vi "Disabled - Data Logger (SubVI).vi"(4 "Data Acquisition Array":string[][](array[string]), 7 "Header Names Input":string[](array[string]), 8 "File Index In":i32, 9 "was teleop Input?":bool, 10 "File Name":string, 11 "Path":string="/home/lvuser/Data/") -> (0 "File Index Out":i32, 2 "File Name Out":string, 3 "Was in Teleop Ouput?":bool)   [LabVIEW 2019]
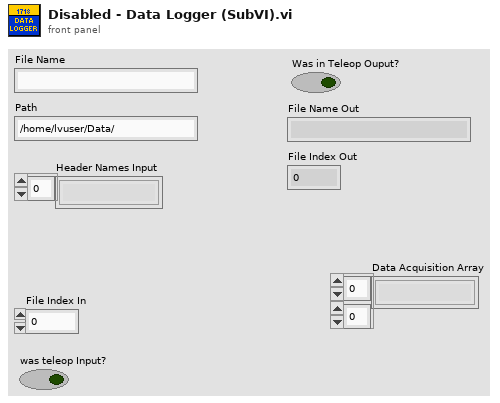
[diagram p1: front panel]
types:
  T1 = enum16{"open", "replace", "create", "open or create", "replace or create", "replace or create with confirmation"}
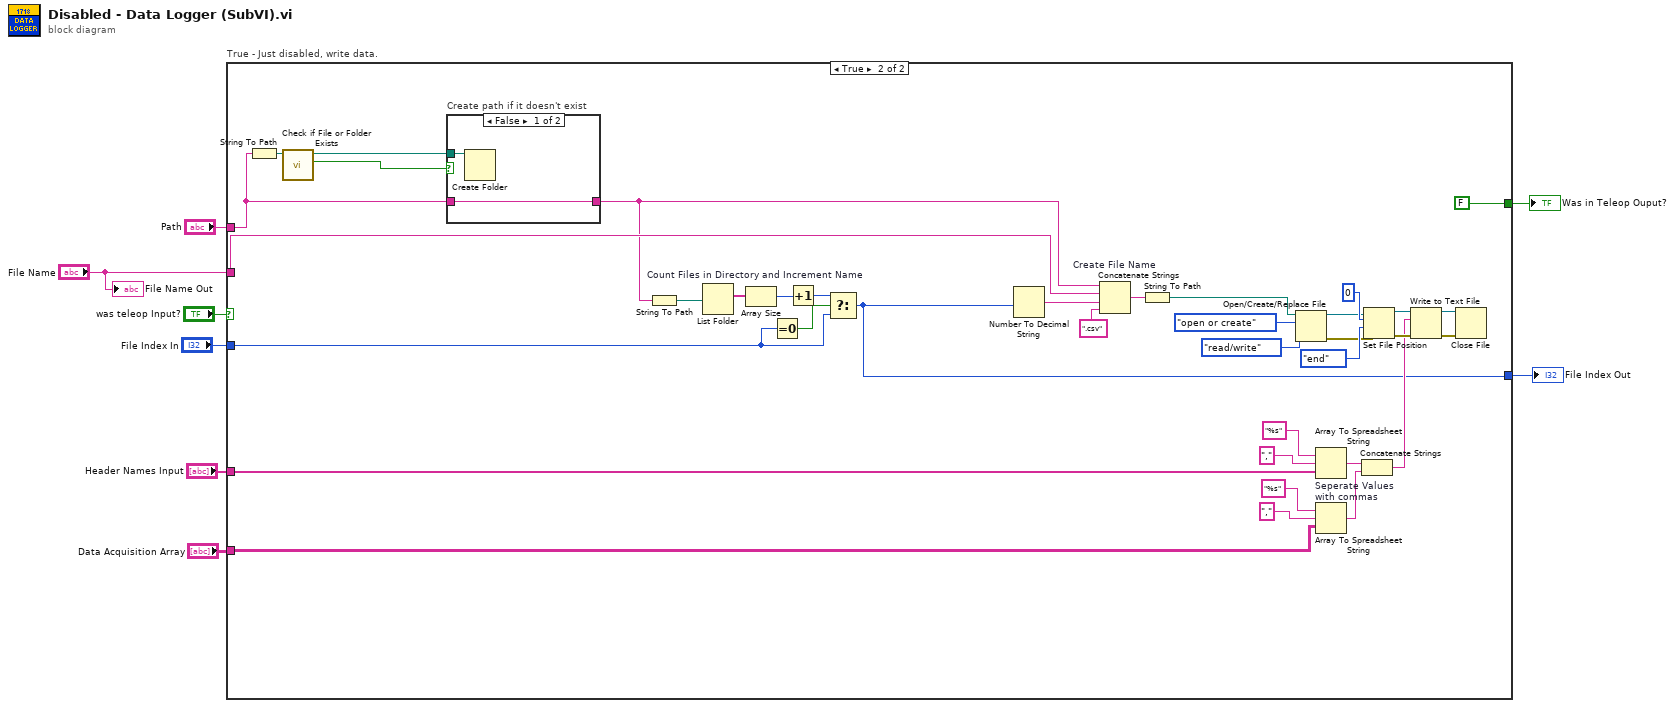
[diagram p0: block diagram]
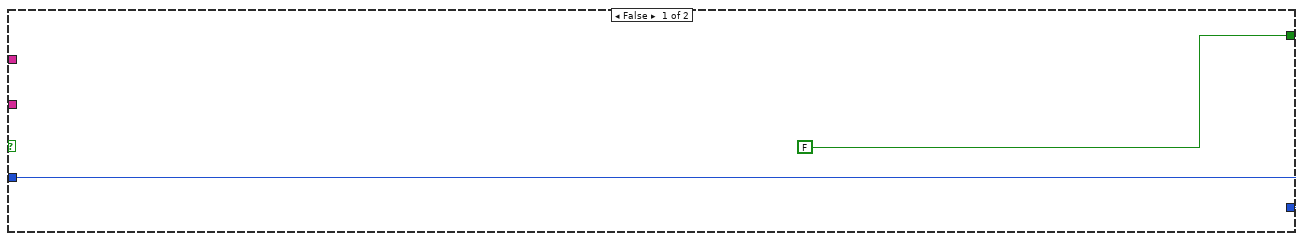
[diagram p2: hidden frame]
diagram:
  n1 = case "True - Just disabled, write data." shown="True" "was teleop Input?" {
    tunnel: [FALSE FALSE] -> w5
    tunnel: "Data Acquisition Array" -> [_ w11]
    tunnel: "Header Names Input" -> [_ w33]
    tunnel: "Path" -> [_ w18]
    tunnel: "File Name" -> [_ w29]
    tunnel: "File Index In" -> [w9 w13]
    tunnel: [w9 w12] -> w2
    frame False {
    }
    frame True {
      n2 = String To Path(string=w18) -> (path=w19:path)
      n3 = call <vilib>:"Check if File or Folder Exists.vi"("path"=w19) -> ("file or folder exists?"=w20:bool, "dup path"=w16:path)  [unwired: 8 in, 1 out]
      n4 = case "Create path if it doesn't exist" shown="False" w20 {
        tunnel: w16 -> [w49 _]
        tunnel: w18 -> [w48 w50]
        tunnel: [w48 w50] -> w17
        frame False {
          n5 = Create Folder(path (use dialog)=w49) -> ()  [unwired: 2 in, 3 out]
        }
        frame True {
        }
      }
      n6 = String To Path(string=w17) -> (path=w31:path)
      n7 = List Folder "Count Files in Directory and Increment Name"(path=w31) -> (filenames=w32:string[])  [unwired: 1 in, 5 out]
      n8 = Array Size(array=w32) -> (size(s)=w28:i32)
      n9 = Equal To 0?(x=w13) -> (x = 0?=w15:bool)
      n10 = Increment(x=w28) -> (x+1=w14:i32)
      n11 = Select(t=w14, s=w15, f=w13) -> (s? t:f=w12:i32)
      n12 = Number To Decimal String(number=w12) -> (decimal integer string=w27:string)  [unwired: 1 in]
      n13 = Concatenate Strings "Create File Name"(w17, w29, w27, ".csv" ("string")) -> (w26:string)
      n14 = String To Path(string=w26) -> (path=w25:path)
      n15 = Open/Create/Replace File(file path (use dialog)=w25, operation (0:open)=T1."open or create", access (0:read/write)=enum16{"read/write", "read-only", "write-only"}."read/write") -> (refnum out=w24:refnum<file>, error out=w23:errorcluster)  [unwired: 3 in, 1 out]
      n16 = Array To Spreadsheet String "Seperate Values\nwith commas"(delimiter (Tab)=",", array=w33, 3:"%s" ("format string")) -> (spreadsheet string=w34:string)
      n17 = Array To Spreadsheet String(delimiter (Tab)=",", array=w11, 3:"%s" ("format string")) -> (spreadsheet string=w37:string)
      n18 = Concatenate Strings(w34, w37) -> (w38:string)
      n19 = Set File Position(offset (in bytes) (0)=i64 0, refnum=w24, from (0:start)=enum16{"start", "end", "current"}."end", error in=w23) -> (refnum out=w47:refnum<file>, error out=w45:errorcluster)
      n20 = Write to Text File(file (use dialog)=w47, text=w38, error in=w45) -> (refnum out=w46:refnum<file>, error out=w44:errorcluster)  [unwired: 1 in, 1 out]
      n21 = Close File(refnum=w46, error in=w44) -> ()  [unwired: 2 out]
    }
  }
  "Was in Teleop Ouput?" <- w5
  "File Index Out" <- w2
  "File Name Out" <- "File Name"
